vi "Envio dados HTTP LabVIEW Gás coz.vi"(1 "valorAnalogicoTemp":dbl) -> ()   [LabVIEW 2020]
uses:
  <vilib>/httpClient/LabVIEWHTTPClient.lvlib
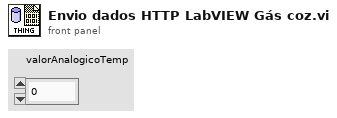
[diagram p1: front panel]
types:
  T1 = typedef "LabVIEWHTTPClient.lvlib/ClientHandle.ctl" = refnum<k1>
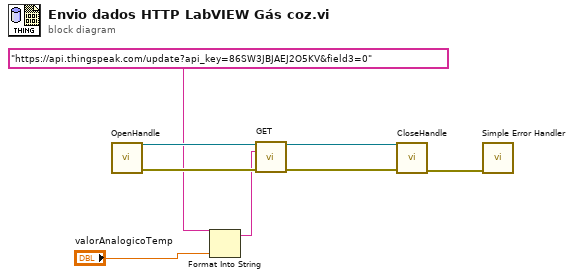
[diagram p0: block diagram]
diagram:
  n1 = call <vilib>:"OpenHandle.vi"() -> ("client handle out"=w7:T1, "error out"=w8:errorcluster)  [unwired: 14 in]
  n2 = Format Into String "Format Into String"(initial string="https://api.thingspeak.com/update?api_key=86SW3JBJAEJ2O5KV&field3=0", "valorAnalogicoTemp") -> (resulting string=w2:string)  [unwired: 2 in, 1 out]
  n3 = call <vilib>:"GET.vi"("client handle"=w7, "url"=w2, "error in (no error)"=w8) -> ("client handle out"=w6:T1, "error out"=w5:errorcluster)  [unwired: 9 in, 2 out]
  n4 = call <vilib>:"CloseHandle.vi"("client handle"=w6, "error in (no error)"=w5) -> ("error out"=w4:errorcluster)  [unwired: 13 in]
  n5 = call <vilib>:"Simple Error Handler.vi"("error in (no error)"=w4) -> ()  [unwired: 4 in, 5 out]
